vi "Send Camera Optics Diagnostics_RC.vi"(7 "Message Priority (Normal)":T2=enum."Normal", 8 "error in (no error)":errorcluster, 10 "Light Camera Info":T1, 11 "Message Enqueuer":refnum<class "Message Enqueuer.lvclass">) -> (0 "error out":errorcluster, 3 "Message Enqueuer out":refnum<class "Message Enqueuer.lvclass">)   [LabVIEW 2019, in "Camera Optics Diagnostics_RC Msg.lvclass"]
doc: "This VI sends the message to an actor."
uses:
  Camera Optics Diagnostics_RC Msg.lvclass
  <vilib>/ActorFramework/Message Enqueuer/Message Enqueuer.lvclass
  C:/Program Files/National Instruments/LabVIEW 2019/vi.lib/ActorFramework/Message/Message.lvclass
  <vilib>/ActorFramework/Message Enqueuer/Message Priority.ctl
  Common/Controls/Camera Optics Diagnostics.ctl
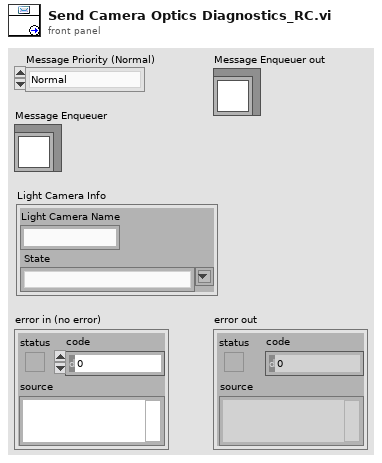
[diagram p1: front panel]
types:
  T1 = typedef "Camera Optics Diagnostics.ctl" = cluster{"Light Camera Name":string, " State":string}
  T2 = typedef "Actor Framework.lvlib/Message Enqueuer.lvclass/Message Priority.ctl" = enum16{"Low", "Normal", "High"}
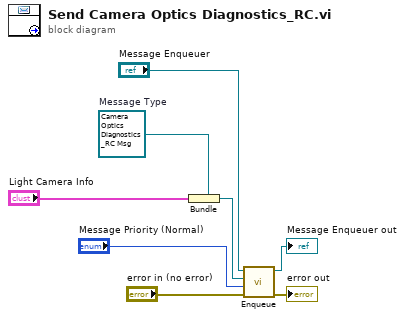
[diagram p0: block diagram]
diagram:
  w5 = refnum<class "Camera Optics Diagnostics_RC Msg.lvclass"> refnum  # Message Type
  n1 = Bundle(cluster=w5, "Light Camera Info") -> (w4:refnum<class "Camera Optics Diagnostics_RC Msg.lvclass">)
  n2 = call <vilib>:"Enqueue.vi"("error in (no error)"="error in (no error)", "Message Priority (Normal)"="Message Priority (Normal)", "Message"=w4, "Message Enqueuer in"="Message Enqueuer") -> ("error out"=→"error out":errorcluster, "Message Enqueuer out"=→"Message Enqueuer out":refnum<class "Message Enqueuer.lvclass">)  [unwired: 6 in]
